vi "sting_to_char.vi"(1 "String":string) -> (0 "Char":string)   [LabVIEW 2010]
panel:
  out "unsigned byte array":u8[](array[numeric])
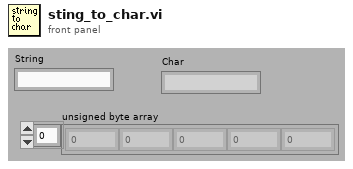
[diagram p1: front panel]
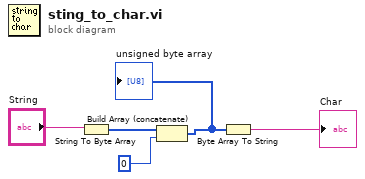
[diagram p0: block diagram]
diagram:
  n1 = String To Byte Array(string="String") -> (unsigned byte array=w4:u8[])
  n2 = Build Array (concatenate)(w4, u8 0) -> (w1:u8[])
  "unsigned byte array" <- w1
  n3 = Byte Array To String(unsigned byte array=w1) -> (string=→"Char":string)
